vi "Checkers Credits.vi"() -> ()   [LabVIEW 2014]
panel:
  in  "MAIN MENU":bool
  # "CREDITS:"
  # "PROGRAMMERS:"
  # "RITESH MISRA, DANIEL SOKOLOWSKI"
  # "LABVIEW INSTRUCTOR:"
  # "DR. BRIAN MOYER"
  # "MUSIC:"
  # "MENU MUSIC..............................................GYMNOPEDIE #1\n                                                                            BY: ERIC SATIE"
  # "GAME MUSIC...........................................................PALLADIO\n                                                                      BY: KARL JENKINS"
  # "ILLUSTRATIONS:"
  # "CHECKERBOARD...............http://wordaligned.org/images/chessboard-magick.png"
  # "SOFTWARE:"
  # "LabVIEW 2016, STUDENT EDITION, BY NATIONAL INSTRUMENTS"
  # "SPECIAL THANKS TO:"
  # "Bill Gates\nTim Berners-Lee\nOur Parents\nAll Higher Beings, and/or Nature\nDr. Budny\nDr. Patzer\nObama\nFormula nodes\n & mangoes (the fruit)"
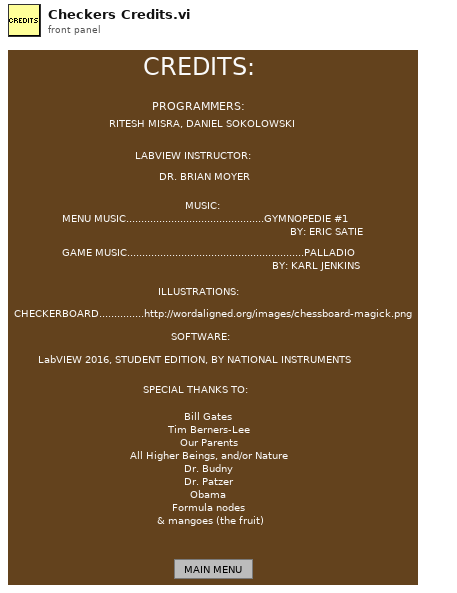
[diagram p1: front panel]
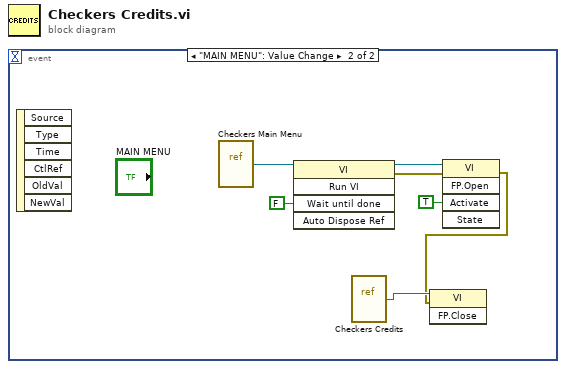
[diagram p0: block diagram]
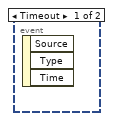
[diagram p2: hidden frame]
diagram:
  n1 = event shown="[1] \"MAIN MENU\": Value Change" {
    selector: _ -> [_ _]
    dyn-events: _ -> [_ _]
    timeout: _ -> [_ _]
    event Timeout {
      n2 = event-data() -> ()  [unwired: 1 in, 3 out]
    }
    event "MAIN MENU": Value Change {
      n3 = event-data() -> ()  [unwired: 1 in, 6 out]
      n4 = vi-ref "Checkers Main Menu.vi"() -> (w7:refnum<vi>)
      n5 = invoke class="VI" method="Run VI"(reference=w7, "Wait until done"=FALSE ("Wait Until Done")) -> (reference out=w6:refnum<vi>, error out=w5:errorcluster)  [unwired: 3 in, 3 out]
      n6 = vi-ref "Checkers Credits.vi"() -> (w2:refnum<vi>)
      n7 = invoke class="VI" method="FP.Open"(reference=w6, error in=w5, "Activate"=TRUE ("Activate?")) -> (error out=w1:errorcluster)  [unwired: 2 in, 4 out]
      n8 = invoke class="VI" method="FP.Close"(reference=w2, error in=w1) -> ()  [unwired: 1 in, 3 out]
    }
  }
